vi "Is Internal Mechanical Shutter.vi"(11 "InternalShutter":i32) -> (2 "function return":u32, 3 "InternalShutter out":i32)   [LabVIEW 2018, in "AndorSDK.lvlib"]
doc: "EXPNETTYPE unsigned int WINAPI IsInternalMechanicalShutter(int * InternalShutter);"
uses:
  AndorSDK.lvlib
  ATMCD32D.dll
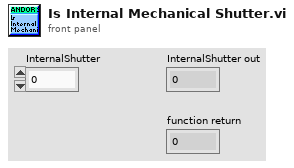
[diagram p1: front panel]
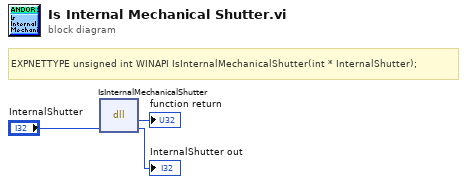
[diagram p0: block diagram]
diagram:
  # "EXPNETTYPE unsigned int WINAPI IsInternalMechanicalShutter(int * InternalShutter);"
  n1 = dll-call lib="PTH2babs E\nPersönliches02 - Arbeit03-HiwijobsLabviewCodelibANDOR\tAndor SDK\nATMCD32D.*" fn="IsInternalMechanicalShutter"("InternalShutter"="InternalShutter") -> (→"function return":u32, "InternalShutter"=→"InternalShutter out":i32)  [unwired: 3 in, 2 out]
